vi "S2C_PCIe7841_Poly_TestBed.vi"() -> ()   [LabVIEW 2015]
uses:
  Typedefs/S2C_PCIe7841_Type_Connector.ctl
  Typedefs/S2C_PCIe7841_Type_Port.ctl
  Typedefs/S2C_PCIe7841_Type_Audio.ctl
  Typedefs/S2C_PCIe7841_Type_HandSwitchWr.ctl
  Typedefs/S2C_PCIe7841_Type_HomerWr.ctl
  Typedefs/S2C_PCIe7841_Type_LxfWr.ctl
  Typedefs/S2C_PCIe7841_Type_HomerRd.ctl
  Typedefs/S2C_PCIe7841_Type_PathRelayWr.ctl
  Typedefs/S2C_PCIe7841_Type_Reserved.ctl
  Typedefs/S2C_PCIe7841_Type_Triverse.ctl
  Typedefs/S2C_PCIe7841_Type_VlacWr.ctl
  Typedefs/S2C_PCIe7841_Type_RemRd.ctl
  Typedefs/S2C_PCIe7841_Type_RemWr.ctl
  Typedefs/S2C_PCIe7841_Type_AnalogWr.ctl
  Typedefs/S2C_PCIe7841_Type_AnalogRd.ctl
  S2C_PCIe7841_Poly_AudioWrite.vi
  S2C_PCIe7841_Poly_AudioRead.vi
  S2C_PCIe7841_Poly_HandSwitchWrite.vi
  S2C_PCIe7841_Poly_HandSwitchRead.vi
  S2C_PCIe7841_Poly_HomerWrite.vi
  S2C_PCIe7841_Poly_HomerRead.vi
  S2C_PCIe7841_Poly_LxfWrite.vi
  S2C_PCIe7841_Poly_LxfRead.vi
  S2C_PCIe7841_Poly_PalletRead.vi
  S2C_PCIe7841_Poly_RelayPathWrite.vi
  S2C_PCIe7841_Poly_RelayPathRead.vi
  S2C_PCIe7841_Poly_RemWrite.vi
  S2C_PCIe7841_Poly_RemRead.vi
  S2C_PCIe7841_Poly_ReservedWrite.vi
  S2C_PCIe7841_Poly_ReservedRead.vi
  S2C_PCIe7841_Poly_SmokeEvacRead.vi
  S2C_PCIe7841_Poly_TriverseWrite.vi
  S2C_PCIe7841_Poly_TriverseRead.vi
  S2C_PCIe7841_Poly_VlacWrite.vi
  S2C_PCIe7841_Poly_VlacRead.vi
  S2C_PCIe7841_Poly_AnalogWrite.vi
  S2C_PCIe7841_Poly_AnalogRead.vi
  S2C_PCIe7841_Poly_PortWrite.vi
  S2C_PCIe7841_Poly_PortRead.vi
panel:
  out "Error Out":errorcluster
  in  "Error In":errorcluster
  out "Response":T1
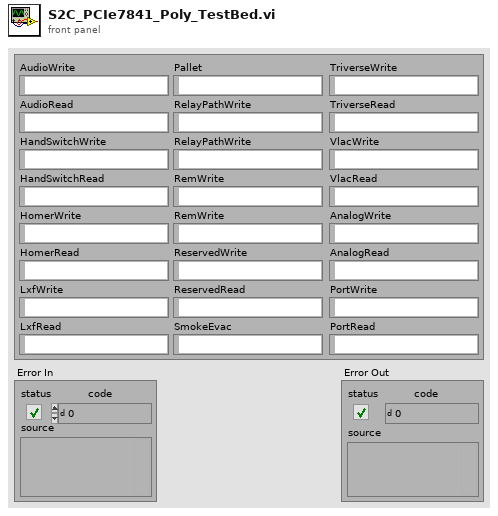
[diagram p1: front panel]
types:
  T1 = cluster{"AudioWrite":string, "AudioRead":string, "HandSwitchWrite":string, "HandSwitchRead":string, "HomerWrite":string, "HomerRead":string, "LxfWrite":string, "LxfRead":string, "Pallet":string, "RelayPathWrite":string, "RelayPathWrite":string, "RemWrite":string, "RemWrite":string, "ReservedWrite":string, "ReservedRead":string, "SmokeEvac":string, "TriverseWrite":string, "TriverseRead":string, "VlacWrite":string, "VlacRead":string, "AnalogWrite":string, "AnalogRead":string, "PortWrite":string, "PortRead":string}
  T2 = typedef "S2C_PCIe7841_Type_AnalogRd.ctl" = u16
  T3 = typedef "S2C_PCIe7841_Type_AnalogWr.ctl" = u16
  T4 = typedef "S2C_PCIe7841_Type_RemWr.ctl" = string
  T5 = typedef "S2C_PCIe7841_Type_RemRd.ctl" = string
  T6 = typedef "S2C_PCIe7841_Type_VlacWr.ctl" = string
  T7 = typedef "S2C_PCIe7841_Type_Triverse.ctl" = string
  T8 = typedef "S2C_PCIe7841_Type_Reserved.ctl" = string
  T9 = typedef "S2C_PCIe7841_Type_PathRelayWr.ctl" = string
  T10 = typedef "S2C_PCIe7841_Type_HomerRd.ctl" = string
  T11 = typedef "S2C_PCIe7841_Type_LxfWr.ctl" = string
  T12 = typedef "S2C_PCIe7841_Type_HomerWr.ctl" = string
  T13 = typedef "S2C_PCIe7841_Type_HandSwitchWr.ctl" = string
  T14 = typedef "S2C_PCIe7841_Type_Audio.ctl" = string
  T15 = typedef "S2C_PCIe7841_Type_Connector.ctl" = u16
  T16 = typedef "S2C_PCIe7841_Type_Port.ctl" = u16
  T17 = cluster{"Connector":T15, "Port":T16, "Data":string}
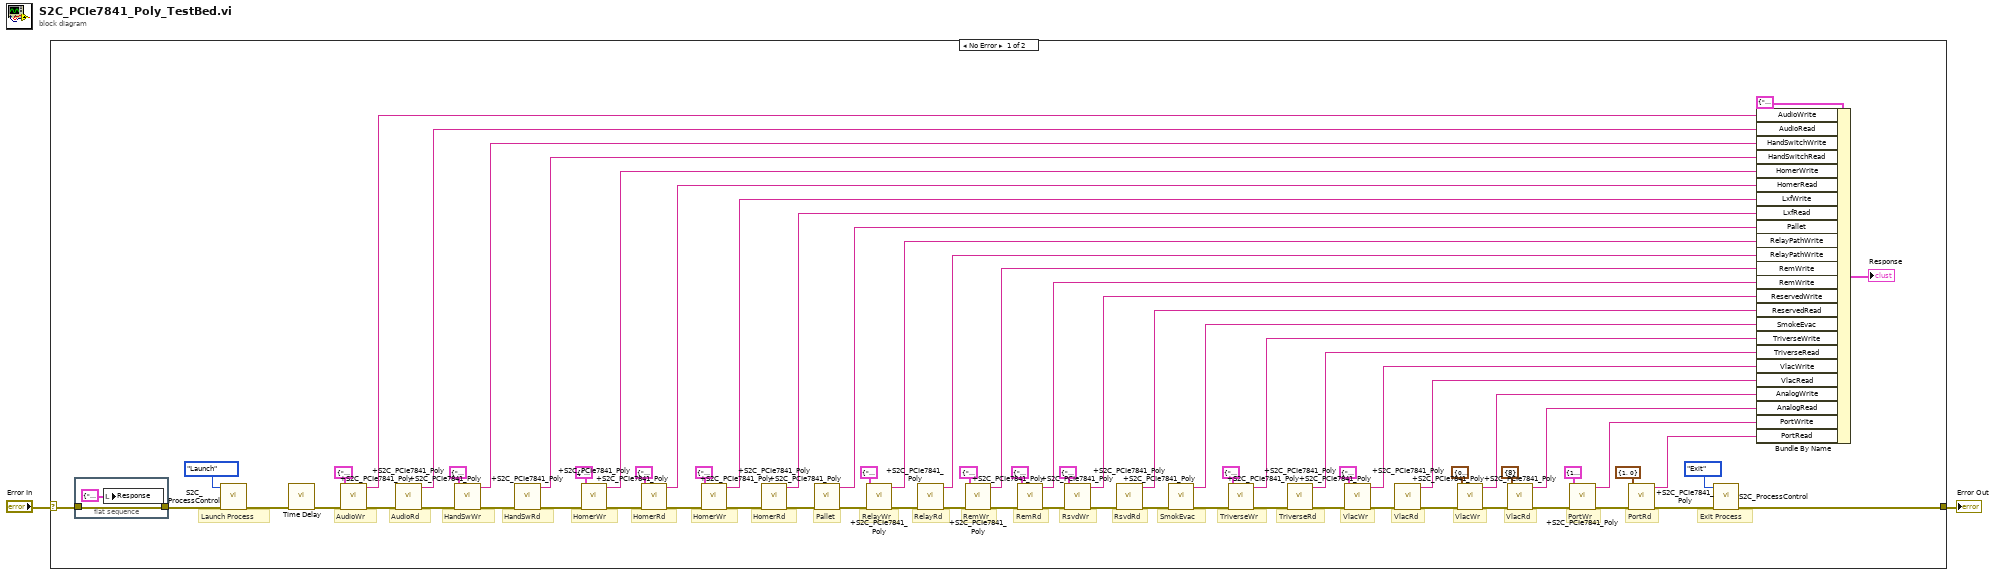
[diagram p0: block diagram]
diagram:
  n1 = case shown="No Error" "Error In" {
    selector: "Error In" -> [w69 w77]
    tunnel: [w71 w77] -> w1
    frame No Error {
      # "VlacRd"
      # "VlacWr"
      # "VlacRd"
      # "VlacWr"
      # "TriverseRd"
      # "TriverseWr"
      # "SmokEvac"
      # "RsvdRd"
      # "RsvdWr"
      # "RemRd"
      # "RemWr"
      # "RelayRd"
      # "RelayWr"
      # "Pallet"
      # "HomerRd"
      # "HomerWr"
      # "HomerRd"
      # "HomerWr"
      # "HandSwRd"
      # "HandSwWr"
      # "AudioRd"
      # "AudioWr"
      # "PortRd"
      # "PortWr"
      # "Exit Process"
      # "Launch Process"
      n2 = flat-sequence {
        tunnel: w69 -> [w76]
        tunnel: [w76] -> w68
        frame #0 {
          n3 = local write "Response"(T1 {"AudioWrite"="", "AudioRead"="", "HandSwitchWrite"="", "HandSwitchRead"="", "HomerWrite"="", "HomerRead"="", "LxfWrite"="", "LxfRead"="", "Pallet"="", "RelayPathWrite"="", "RelayPathWrite"="", "RemWrite"="", "RemWrite"="", "ReservedWrite"="", "ReservedRead"="", "SmokeEvac"="", "TriverseWrite"="", "TriverseRead"="", "VlacWrite"="", "VlacRead"="", "AnalogWrite"="", "AnalogRead"="", "PortWrite"="", "PortRead"=""} ("Response")) -> ()
        }
      }
      n4 = call "S2C_ProcessControl.vi"("Error In"=w68, "Action"=enum16{"Launch", "Exit"}."Launch") -> ("Error Out"=w73:errorcluster)  [unwired: 9 in]
      n5 = call "Time Delay"("error in (no error)"=w73) -> ("error out"=w66:errorcluster)  [unwired: 10 in]
      n6 = call-poly "+S2C_PCIe7841_Poly.vi"("Error In"=w66, "Audio"=cluster{"Audio":T14, "State":bool} {"Audio"="006", "State"=TRUE}) -> ("Error Out"=w36:errorcluster, "Response"=w70:string)  [unwired: 8 in]
      n7 = call-poly "+S2C_PCIe7841_Poly.vi"("Error In"=w36) -> ("Error Out"=w35:errorcluster, "Response"=w67:string)  [unwired: 9 in]
      n8 = call-poly "+S2C_PCIe7841_Poly.vi"("Error In"=w35, "HandSwitch"=cluster{"HandSwitch":T13, "State":bool} {"HandSwitch"="220", "State"=TRUE}) -> ("Error Out"=w34:errorcluster, "Response"=w65:string)  [unwired: 8 in]
      n9 = call-poly "+S2C_PCIe7841_Poly.vi"("Error In"=w34) -> ("Error Out"=w31:errorcluster, "Response"=w64:string)  [unwired: 9 in]
      n10 = call-poly "+S2C_PCIe7841_Poly.vi"("Error In"=w31, "Homer"=cluster{"Homer":T12, "State":bool} {"Homer"="117", "State"=TRUE}) -> ("Error Out"=w33:errorcluster, "Response"=w63:string)  [unwired: 8 in]
      n11 = call-poly "+S2C_PCIe7841_Poly.vi"("Error In"=w33, "Homer"=cluster{"Homer":T10} {"Homer"="117"}) -> ("Error Out"=w30:errorcluster, "Response"=w62:string)  [unwired: 8 in]
      n12 = call-poly "+S2C_PCIe7841_Poly.vi"("Error In"=w30, "LXF"=cluster{"LXF":T11, "State":bool} {"LXF"="225", "State"=TRUE}) -> ("Error Out"=w32:errorcluster, "Response"=w61:string)  [unwired: 8 in]
      n13 = call-poly "+S2C_PCIe7841_Poly.vi"("Error In"=w32) -> ("Error Out"=w22:errorcluster, "Response"=w60:string)  [unwired: 9 in]
      n14 = call-poly "+S2C_PCIe7841_Poly.vi"("Error In"=w22) -> ("Error Out"=w24:errorcluster, "Response"=w59:string)  [unwired: 9 in]
      n15 = call-poly "+S2C_PCIe7841_Poly.vi"("Error In"=w24, "RelayPath"=cluster{"RelayPath":T9, "State":bool} {"RelayPath"="110", "State"=TRUE}) -> ("Error Out"=w23:errorcluster, "Response"=w58:string)  [unwired: 8 in]
      n16 = call-poly "+S2C_PCIe7841_Poly.vi"("Error In"=w23) -> ("Error Out"=w20:errorcluster, "Response"=w57:string)  [unwired: 9 in]
      n17 = call-poly "+S2C_PCIe7841_Poly.vi"("Error In"=w20, "REM"=cluster{"REM":T4, "State":bool} {"REM"="120", "State"=TRUE}) -> ("Error Out"=w21:errorcluster, "Response"=w56:string)  [unwired: 8 in]
      n18 = call-poly "+S2C_PCIe7841_Poly.vi"("Error In"=w21, "REM"=cluster{"REM":T5} {"REM"="120"}) -> ("Error Out"=w18:errorcluster, "Response"=w55:string)  [unwired: 8 in]
      n19 = call-poly "+S2C_PCIe7841_Poly.vi"("Error In"=w18, "Reserved"=cluster{"Reserved":T8, "State":bool} {"Reserved"="244", "State"=TRUE}) -> ("Error Out"=w19:errorcluster, "Response"=w54:string)  [unwired: 8 in]
      n20 = call-poly "+S2C_PCIe7841_Poly.vi"("Error In"=w19) -> ("Error Out"=w16:errorcluster, "Response"=w53:string)  [unwired: 9 in]
      n21 = call-poly "+S2C_PCIe7841_Poly.vi"("Error In"=w16) -> ("Error Out"=w17:errorcluster, "Response"=w52:string)  [unwired: 9 in]
      n22 = call-poly "+S2C_PCIe7841_Poly.vi"("Error In"=w17, "Triverse"=cluster{"Triverse":T7, "State":bool} {"Triverse"="201", "State"=TRUE}) -> ("Error Out"=w15:errorcluster, "Response"=w51:string)  [unwired: 8 in]
      n23 = call-poly "+S2C_PCIe7841_Poly.vi"("Error In"=w15) -> ("Error Out"=w13:errorcluster, "Response"=w50:string)  [unwired: 9 in]
      n24 = call-poly "+S2C_PCIe7841_Poly.vi"("Error In"=w13, "VLAC"=cluster{"VLAC":T6, "State":bool} {"VLAC"="144", "State"=TRUE}) -> ("Error Out"=w14:errorcluster, "Response"=w49:string)  [unwired: 8 in]
      n25 = call-poly "+S2C_PCIe7841_Poly.vi"("Error In"=w14) -> ("Error Out"=w5:errorcluster, "Response"=w48:string)  [unwired: 9 in]
      n26 = call-poly "+S2C_PCIe7841_Poly.vi"("Error In"=w5, "Analog IO"=cluster{"Analog Output":T3, "Output Value":dbl} {"Analog Output"=0, "Output Value"=1.2345}) -> ("Error Out"=w6:errorcluster, "Response"=w47:string)  [unwired: 8 in]
      n27 = call-poly "+S2C_PCIe7841_Poly.vi"("Error In"=w6, "Analog IO"=cluster{"Analog IO":T2} {"Analog IO"=8}) -> ("Error Out"=w45:errorcluster, "Response"=w46:string)  [unwired: 8 in]
      n28 = call-poly "+S2C_PCIe7841_Poly.vi"("Error In"=w45, "WritePort"=T17 {"Connector"=1, "Port"=0, "Data"="10101010"}) -> ("Error Out"=w39:errorcluster, "Response"=w44:string)  [unwired: 8 in]
      n29 = call-poly "+S2C_PCIe7841_Poly.vi"("Error In"=w39, "PortRead"=cluster{"Connector":T15, "Port":T16} {"Connector"=1, "Port"=0}) -> ("Error Out"=w38:errorcluster, "Response"=w41:string)  [unwired: 8 in]
      n30 = call "S2C_ProcessControl.vi"("Error In"=w38, "Action"=enum16{"Launch", "Exit"}."Exit") -> ("Error Out"=w71:errorcluster)  [unwired: 9 in]
      n31 = Bundle By Name(cluster=T1 {"AudioWrite"="", "AudioRead"="", "HandSwitchWrite"="", "HandSwitchRead"="", "HomerWrite"="", "HomerRead"="", "LxfWrite"="", "LxfRead"="", "Pallet"="", "RelayPathWrite"="", "RelayPathWrite"="", "RemWrite"="", "RemWrite"="", "ReservedWrite"="", "ReservedRead"="", "SmokeEvac"="", "TriverseWrite"="", "TriverseRead"="", "VlacWrite"="", "VlacRead"="", "AnalogWrite"="", "AnalogRead"="", "PortWrite"="", "PortRead"=""} ("Response"), "AudioWrite"=w70, "AudioRead"=w67, "HandSwitchWrite"=w65, "HandSwitchRead"=w64, "HomerWrite"=w63, "HomerRead"=w62, "LxfWrite"=w61, "LxfRead"=w60, "Pallet"=w59, "RelayPathWrite"=w58, "RelayPathWrite"=w57, "RemWrite"=w56, "RemWrite"=w55, "ReservedWrite"=w54, "ReservedRead"=w53, "SmokeEvac"=w52, "TriverseWrite"=w51, "TriverseRead"=w50, "VlacWrite"=w49, "VlacRead"=w48, "AnalogWrite"=w47, "AnalogRead"=w46, "PortWrite"=w44, "PortRead"=w41) -> (→"Response":T1)
    }
    frame Error {
    }
  }
  "Error Out" <- w1
